vi "Create Publish Data Events.vi"(8 "error in (no error)":errorcluster, 11 "UserEvents in":refnum<class "UserEvents.lvclass">) -> (0 "error out":errorcluster, 3 "UserEvents out":refnum<class "UserEvents.lvclass">)   [LabVIEW 2015, in "UserEvents.lvclass"]
uses:
  UserEvents.lvclass
  Typedefs/State Types.ctl
  Typedefs/Scan Progress.ctl
  <userlib>/Common/ILC/Typedefs/Outputs.ctl
  <userlib>/Common/ILC/Typedefs/ADC Eng.ctl
  UserEvents.lvclass/UserEvents.ctl
  Typedefs/FAMT Typedefs.lvlib
  <userlib>/Common/ILC/Typedefs/ILCTypedefs.lvlib
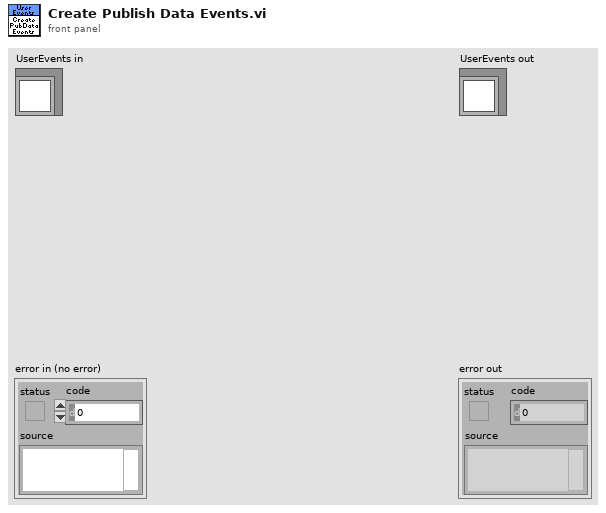
[diagram p1: front panel]
types:
  T1 = typedef "ILCCommon.lvlib/ILCTypedefs.lvlib/ADC Eng.ctl" = cluster{"Ch1":dbl[unit], "Ch2":dbl[unit], "Ch3":dbl[unit], "Ch4":dbl[unit]}
  T2 = typedef "ILCCommon.lvlib/ILCTypedefs.lvlib/Outputs.ctl" = cluster{"Step & Direction":i16, "Blower RPM":u8, "PWM (SSR)":u8, "Ch1":u16, "Ch2":u16, "Ch3":u16, "Ch4":u16}
  T3 = typedef "FAMT Typedefs.lvlib/Scan Progress.ctl" = cluster{"Waveform Step":u16, "Axial Demand":dbl, "Lateral Demand":dbl, "FC1 Demand":dbl, "FC2 Demand":dbl, "FC1 Measured Force":dbl[unit], "FC2 Measured Force":dbl[unit], "Axial Force":dbl[unit], "Lateral Force":dbl[unit], "A Force":dbl[unit], "B Force":dbl[unit], "C Force":dbl[unit], "D Moment":dbl[unit], "E Moment":dbl[unit], "F Moment":dbl[unit]}
  T4 = typedef "FAMT Typedefs.lvlib/State Types.ctl" = enum16{"Offline State", "Fault State", "Standby State", "Disabled State", "Enabled State", "Wait For User Input State", "Perform Scan State"}
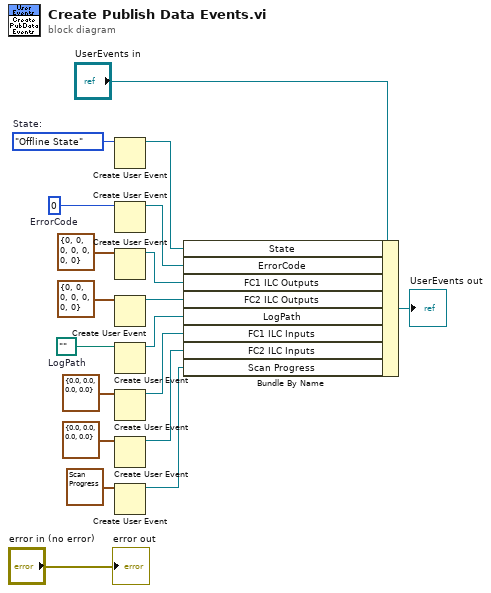
[diagram p0: block diagram]
diagram:
  w10 = path ""  # LogPath
  w15 = 0  # ErrorCode
  w16 = State_Types."Offline State"  # State:
  n1 = Create User Event(user event datatype=w16) -> (user event=w14:refnum<user-event>)  [unwired: 1 in, 1 out]
  n2 = Create User Event(user event datatype=w15) -> (user event=w13:refnum<user-event>)  [unwired: 1 in, 1 out]
  n3 = Create User Event(user event datatype=T2 {"Step & Direction"=0, "Blower RPM"=0, "PWM (SSR)"=0, "Ch1"=0, "Ch2"=0, "Ch3"=0, "Ch4"=0} ("ILC Outputs")) -> (user event=w11:refnum<user-event>)  [unwired: 1 in, 1 out]
  n4 = Create User Event(user event datatype=T2 {"Step & Direction"=0, "Blower RPM"=0, "PWM (SSR)"=0, "Ch1"=0, "Ch2"=0, "Ch3"=0, "Ch4"=0} ("ILC Outputs")) -> (user event=w4:refnum<user-event>)  [unwired: 1 in, 1 out]
  n5 = Create User Event(user event datatype=w10) -> (user event=w9:refnum<user-event>)  [unwired: 1 in, 1 out]
  n6 = Create User Event(user event datatype=T1 {"Ch1"=0.0, "Ch2"=0.0, "Ch3"=0.0, "Ch4"=0.0} ("ILC ADCs Engineering")) -> (user event=w8:refnum<user-event>)  [unwired: 1 in, 1 out]
  n7 = Create User Event(user event datatype=T1 {"Ch1"=0.0, "Ch2"=0.0, "Ch3"=0.0, "Ch4"=0.0} ("ILC ADCs Engineering")) -> (user event=w1:refnum<user-event>)  [unwired: 1 in, 1 out]
  n8 = Create User Event(user event datatype=T3 {"Waveform Step"=0, "Axial Demand"=0.0, "Lateral Demand"=0.0, "FC1 Demand"=0.0, "FC2 Demand"=0.0, "FC1 Measured Force"=0.0, "FC2 Measured Force"=0.0, "Axial Force"=0.0, "Lateral Force"=0.0, "A Force"=0.0, "B Force"=0.0, "C Force"=0.0, "D Moment"=0.0, "E Moment"=0.0, "F Moment"=0.0} ("Chart Data")) -> (user event=w3:refnum<user-event>)  [unwired: 1 in, 1 out]
  n9 = Bundle By Name(cluster="UserEvents in", "State"=w14, "ErrorCode"=w13, "FC1 ILC Outputs"=w11, "FC2 ILC Outputs"=w4, "LogPath"=w9, "FC1 ILC Inputs"=w8, "FC2 ILC Inputs"=w1, "Scan Progress"=w3) -> (→"UserEvents out":refnum<class "UserEvents.lvclass">)
  "error out" <- "error in (no error)"
